vi "Deplacement_Handler.vi"(8 "Error In":errorcluster caption="Entrée d'erreur", 11 "Donnees_Globales_IN":T1) -> (0 "Error Out":errorcluster, 3 "Donnees_Globale_Out":T1)   [LabVIEW 2019]
uses:
  Asc_State_Inputs.ctl
  Etat_Asc.ctl
  <vilib>/Utility/error.llb/Error Cluster From Error Code.vi
  <vilib>/rvi/errors/niLvFpgaAdjustHostInterfaceError.vi
  <vilib>/rvi/interface/nirviReadWriteControl/nirviReadWriteControl.xnode
  NiFpgaLv.dll
  <vilib>/rvi/interface/Simulation/niFpgaSimulationCallBeginRW.vi
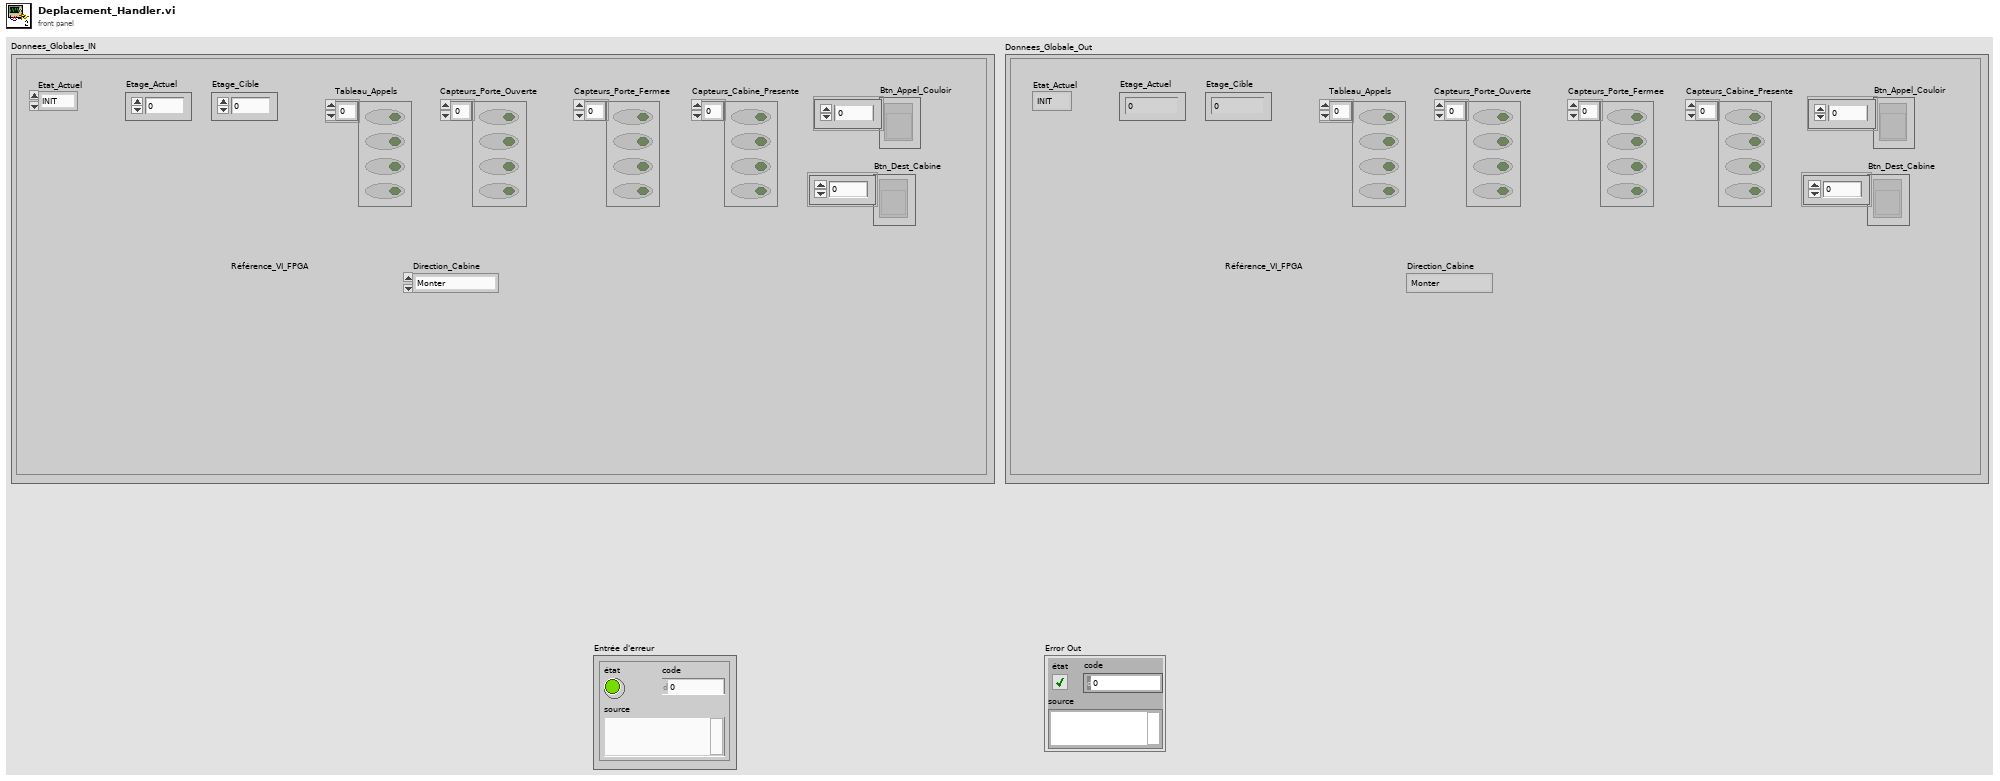
[diagram p1: front panel]
types:
  T1 = typedef "Asc_State_Inputs.ctl" = cluster{"Etage_Actuel":i32, "Etat_Actuel":T2, "Etage_Cible":i32, "Tableau_Appels":bool[], "Capteurs_Porte_Ouverte":bool[], "Capteurs_Porte_Fermee":bool[], "Capteurs_Cabine_Presente":bool[], "Btn_Appel_Couloir":refnum<vi>[], "Btn_Dest_Cabine":refnum<vi>[], "Référence_VI_FPGA":refnum<k20>, "Direction_Cabine":enum16{"Monter", "Descendre", "Arreter"}}
  T2 = typedef "Etat_Asc.ctl" = enum16{"INIT", "REPOS", "DEPLACEMENT", "OUVERTURE_PORTE", "ATTENTE_TEMPO", "FERMETURE_PORTE", "ARRET_URGENCE"}
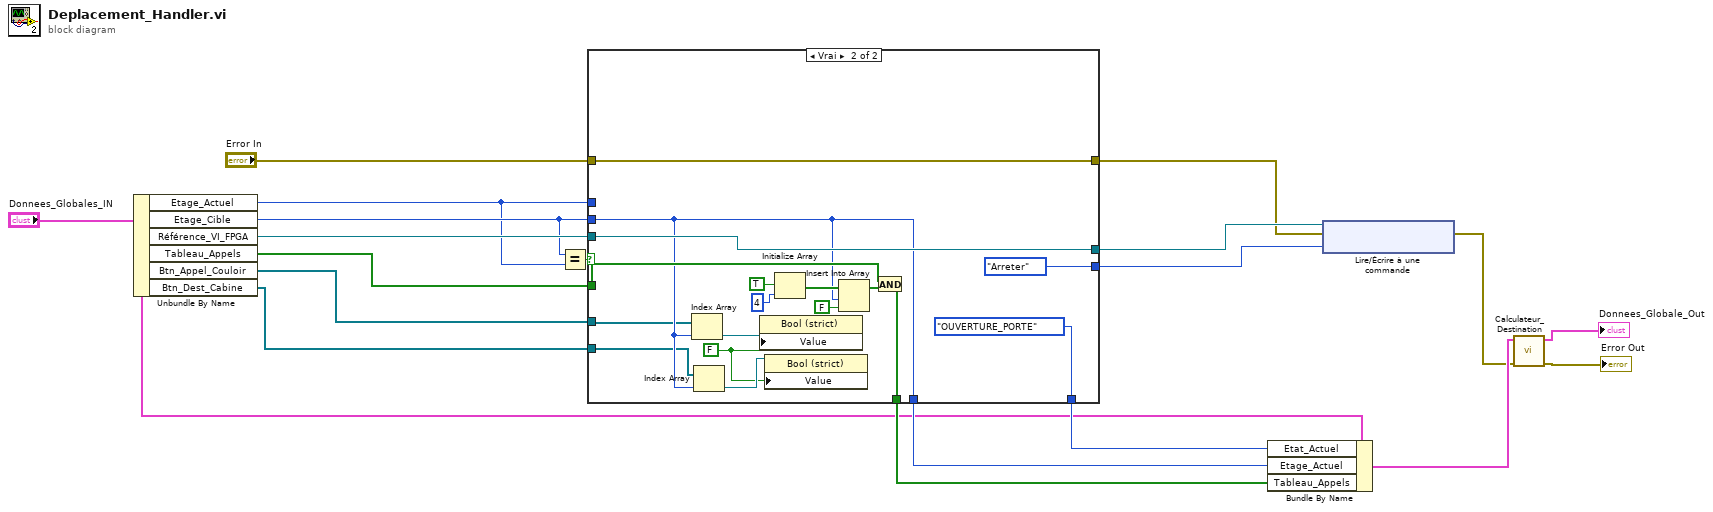
[diagram p0: block diagram]
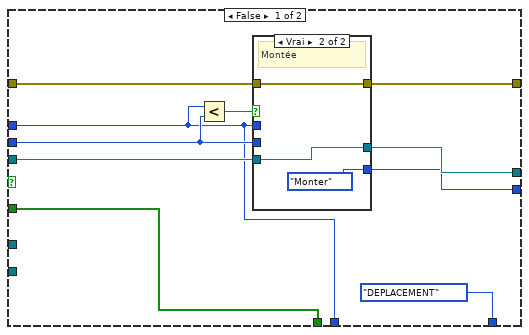
[diagram p2: hidden frame]
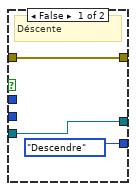
[diagram p3: hidden frame]
diagram:
  n1 = Unbundle By Name("Donnees_Globales_IN") -> ("Etage_Actuel"=w8:i32, "Etage_Cible"=w14:i32, "Référence_VI_FPGA"=w18:refnum<k20>, "Tableau_Appels"=w12:bool[], "Btn_Appel_Couloir"=w10:refnum<vi>[], "Btn_Dest_Cabine"=w9:refnum<vi>[])
  n2 = Equal?(x=w14, y=w8) -> (x = y?=w17:bool)
  n3 = case shown="Vrai" w17 {
    tunnel: w8 -> [w21 _]
    tunnel: w14 -> [w22 w41]
    tunnel: "Error In" -> [w29 w50]
    tunnel: w18 -> [w28 w49]
    tunnel: [w27 w49] -> w16
    tunnel: [w26 w50] -> w5
    tunnel: [w25 enum16{"Monter", "Descendre", "Arreter"}."Arreter" ("CMD_Moteur_Cabine")] -> w7
    tunnel: [Etat_Asc."DEPLACEMENT" ("Etat_Actuel") Etat_Asc."OUVERTURE_PORTE" ("Etat_Actuel")] -> w15
    tunnel: [w21 w41] -> w13
    tunnel: w12 -> [w20 w43]
    tunnel: [w20 w42] -> w11
    tunnel: w10 -> [_ w40]
    tunnel: w9 -> [_ w39]
    frame False {
      n4 = Less?(x=w21, y=w22) -> (x < y?=w23:bool)
      n5 = case shown="Vrai" w23 {
        tunnel: w21 -> [_ _]
        tunnel: w22 -> [_ _]
        tunnel: w29 -> [w30 w33]
        tunnel: w28 -> [w32 w35]
        tunnel: [w32 w35] -> w27
        tunnel: [enum16{"Monter", "Descendre", "Arreter"}."Descendre" ("CMD_Moteur_Cabine") enum16{"Monter", "Descendre", "Arreter"}."Monter" ("CMD_Moteur_Cabine")] -> w25
        tunnel: [w30 w33] -> w26
        frame False {
          # "Déscente"
        }
        frame True {
          # "Montée"
        }
      }
    }
    frame True {
      w36 = FALSE ("Valeur")
      n6 = Index Array(array=w40, index=w41) -> (element=w38:refnum<vi>)
      n7 = Index Array(array=w39, index=w41) -> (element=w37:refnum<vi>)
      n8 = property class="Bool (strict)"(reference=w38, "Value"=w36) -> ()  [unwired: 1 in, 2 out]
      n9 = property class="Bool (strict)"(reference=w37, "Value"=w36) -> ()  [unwired: 1 in, 2 out]
      n10 = Initialize Array(TRUE ("élément"), 4 ("taille de la dimension")) -> (w46:bool[])
      n11 = Insert Into Array(array=w46, index=w41, new element=FALSE ("nouvel élément/sous-tableau")) -> (w44:bool[])
      n12 = And(x=w43, y=w44) -> (x .and. y?=w42:bool[])
    }
  }
  n13 = Bundle By Name(cluster="Donnees_Globales_IN", "Etat_Actuel"=w15, "Etage_Actuel"=w13, "Tableau_Appels"=w11) -> (w4:T1)
  n14 = xnode "Lire/Écrire à une commande"("Référence de VI FPGA en entrée"=w16, "entrée d'erreur"=w5, "CMD_Moteur_Cabine"=w7) -> ("sortie d'erreur"=w3:errorcluster)  [unwired: 1 out]
  n15 = call "Calculateur_Destination.vi"("Error In"=w3, "Donnees_Globales_IN"=w4) -> ("Error Out"=→"Error Out":errorcluster, "Donnees_Globale_Out"=→"Donnees_Globale_Out":T1)  [unwired: 8 in]
